vi "LoadArmPressure_old.vi"(8 "error in (no error)":errorcluster, 9 "SHIFTER DATA":T1, 11 "filepath":path) -> (0 "error out":errorcluster)   [LabVIEW 2013, in "main.lvlib"]
uses:
  main.lvlib
  Components/TypeDef - SHIFTER.ctl
  Components/Dependencies.llb/Exit Event Ref.ctl
  New Design/Controls/Reference Cluster.ctl
  <userlib>/_OpenG.lib/file/file.llb/File Exists - Scalar__ogtk.vi
  <vilib>/Utility/file.llb/Read From Spreadsheet File (DBL).vi
  Components/Dependencies.llb/TLB_Dependencies.lvlib
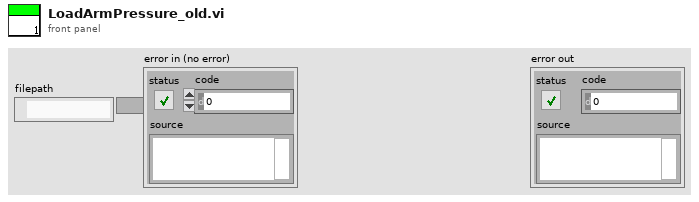
[diagram p1: front panel]
types:
  T1 = typedef "main.lvlib/TypeDef - SHIFTER.ctl" = cluster{"Exit Event":T2, "Terminate Error":errorcluster, "User Parameter Controls":refnum<vi>[], "User Parameters":cluster{"Name":string, "CPR Number":string, "Measuring Type ":string, "Measuring Technique":string, "Measuring Limb":string, "Operator":string, "Doctor":string, "Comment":string, "AdditionalInfo":string, "RightArm":string[][], "LeftArm":string[][], "PalpationRight":string, "PalpationLeft":string, "Puls":dbl, "Temp One":dbl, "Temp Two":dbl, "ActivityBox":bool}, "System Parameters":cluster{"Paper Running?":bool, "GraphSelection":bool, "Date":string, "Active Page":string}, "Data Acquisition":cluster{"Acquisition":bool, "DAQmx Task":refnum<k21>, "DAQmx Error":errorcluster, "Record number":dbl, "RecordPath":path, "AcqDataRef":refnum<vi>, "Duration":timestamp, "Queue":refnum<queue>, "Control?":bool, "RelativeRecordPath":path}, "Reference signal":cluster{"DAQmx  Task ":refnum<k21>, "Monitor":bool, "Events":dbl, "Time":timestamp, "NullEvents":dbl, "RefDataRef":refnum<vi>, "Queue":refnum<queue>}, "Data Process":cluster{"SubpanelRef":refnum<vi>, "ActiveItemTag":string, "Queue":refnum<queue>}, "System Parameter Controls":refnum<vi>[], "Database":cluster{"PatientdataRef":refnum<file>, "PatientdataPath":path, "Blue Pressure":dbl, "Red Pressure":dbl, "ActiveItemTag":string, "Height Adjustment":dbl, "BluePositionArray":dbl[][], "RedPositionArray":dbl[][], "JournalPath":path}, "MWL":cluster{"PatientID":string, "Name":string, "DICOM Info":path, "DICOM Variables":string[], "Worklist":string[][]}, "Control":cluster{"Queue":refnum<queue>, "SignalCluster":cluster{"Pump":bool, "Finger":bool, "Ankle":bool, "Fast Def":bool, "Slow Def":bool, "Init Cal":bool, "Table Pres":bool, "Table":bool}}, "PageMenu":cluster{"VI Reference":refnum<vi>, "Queue":refnum<queue>}, "Profile":cluster{"VI Reference":refnum<vi>, "Queue":refnum<queue>}, "Configuration":cluster{"VI Reference":refnum<vi>, "Queue":refnum<queue>}, "Acquisition":cluster{"VI Reference":refnum<vi>, "Queue":refnum<queue>}, "Data":cluster{"VI Reference":refnum<vi>, "Queue":refnum<queue>}, "Journal":cluster{"VI Reference":refnum<vi>, "Queue":refnum<queue>}, "cRef":T3, "Bluetooth":cluster{"Queue":refnum<queue>, "VI Reference":refnum<vi>}}
  T2 = typedef "main.lvlib/TLB_Dependencies.lvlib/Exit Event Ref.ctl" = refnum<user-event>
  T3 = typedef "main.lvlib/Reference Cluster.ctl" = cluster{"Menu":cluster{"References":cluster{"Stop Acq":refnum<vi>, "MenuExit":refnum<vi>, "MenuStartADC":refnum<vi>, "PersonalInfoString":refnum<vi>, "Profile":refnum<vi>, "Configuration":refnum<vi>, "Acquisition":refnum<vi>, "Data":refnum<vi>, "Journal":refnum<vi>}}, "Profile":cluster{"References":cluster{"Search Patient ID":refnum<vi>, "Name":refnum<vi>, "CommentStr":refnum<vi>, "Listbox Patient ID":refnum<vi>, "ListboxDoctor":refnum<vi>, "ListboxOperator":refnum<vi>, "HospitalName":refnum<vi>, "HospitalDepartment":refnum<vi>, "HospitalAddress":refnum<vi>, "EditHospInfo":refnum<vi>, "Add Patient ID Btn":refnum<vi>, "Query Worklist":refnum<vi>}}, "Configuration":cluster{"References":cluster{"ListboxMeasurementArea":refnum<vi>, "ListboxMeasurementTechnique":refnum<vi>, "ListboxMeasurementMeth":refnum<vi>, "ListboxRightSegmentNr":refnum<vi>, "ListboxLeftSegmentNr":refnum<vi>, "HeightAdjustmentInt":refnum<vi>, "PalpationRight":refnum<vi>, "PalpationLeft":refnum<vi>, "ActivityBox":refnum<vi>}, "New method":cluster{"AddNewMeasurementBtn":refnum<vi>, "Left Time Table":refnum<vi>, "Right Time Table":refnum<vi>}, "Old method":cluster{"LeftArmPressureTable":refnum<vi>, "RightArmPressureTable":refnum<vi>, "SaveArmPressureBtn":refnum<vi>, "Puls":refnum<vi>, "TempTwo":refnum<vi>, "TempOne":refnum<vi>}, "Method":string}, "Acquisition":cluster{"References":cluster{"SegmentAcqString":refnum<vi>, "RingActGraph":refnum<vi>}}, "Data":cluster{"References":cluster{"cmString":refnum<vi>, "AdjustedHeight":refnum<vi>, "Menu":refnum<vi>, "Tangent On/Off":refnum<vi>, "FilterControl":refnum<vi>}}, "Journal":cluster{"References":cluster{"ReportSelection":refnum<vi>, "Data":refnum<vi>, "GenerateReport":refnum<vi>, "Menu":refnum<vi>, "Send To PACS":refnum<vi>}}}
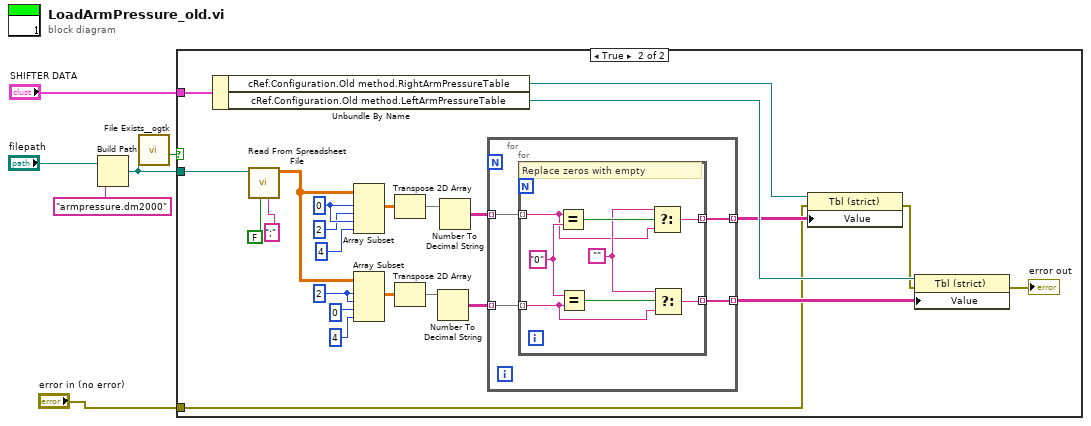
[diagram p0: block diagram]
diagram:
  n1 = Build Path(base path="filepath", name or relative path="armpressure.dm2000") -> (appended path=w2:path)
  n2 = call-poly <userlib>:"File Exists__ogtk.vi"("file path"=w2) -> ("exists"=w4:bool)  [unwired: 6 in, 1 out]
  n3 = case shown="True" w4 {
    tunnel: w2 -> [_ w30]
    tunnel: "SHIFTER DATA" -> [_ w16]
    tunnel: "error in (no error)" -> [_ w8]
    frame False {
    }
    frame True {
      w19 = 2 ("index")
      w27 = 0 ("index")
      n4 = Unbundle By Name(w16) -> ("cRef.Configuration.Old method.RightArmPressureTable"=w15:refnum<vi>, "cRef.Configuration.Old method.LeftArmPressureTable"=w14:refnum<vi>)
      n5 = call-poly <vilib>:"Read From Spreadsheet File.vi"("delimiter (\\t)"=";" ("delimiter (\\t)"), "transpose (no:F)"=FALSE, "file path (dialog if empty)"=w30) -> ("all rows"=w25:dbl[][])  [unwired: 4 in, 4 out]
      n6 = Array Subset(array=w25, index (row)=w27, length (row)=2 ("length"), index (col)=w27, length (col)=4 ("length")) -> (w21:dbl[][])
      n7 = Array Subset(array=w25, index (row)=w19, length (row)=w19, index (col)=0 ("index"), length (col)=4 ("length")) -> (w20:dbl[][])
      n8 = Transpose 2D Array(2D array=w21) -> (transposed array=w18:dbl[][])
      n9 = Transpose 2D Array(2D array=w20) -> (transposed array=w17:dbl[][])
      n10 = Number To Decimal String(number=w17) -> (decimal integer string=w12:string[][])  [unwired: 1 in]
      n11 = Number To Decimal String(number=w18) -> (decimal integer string=w13:string[][])  [unwired: 1 in]
      n12 = for {
        tunnel: w13 -> [w33] mode=indexing
        tunnel: w12 -> [w34] mode=indexing
        tunnel: [w32] -> w11 mode=indexing
        tunnel: [w31] -> w10 mode=indexing
        n13 = for {
          tunnel: w34 -> [w37] mode=indexing
          tunnel: w33 -> [w38] mode=indexing
          tunnel: [w36] -> w32 mode=indexing
          tunnel: [w35] -> w31 mode=indexing
          w39 = ""
          w42 = "0"
          # "Replace zeros with empty"
          n14 = Equal?(x=w38, y=w42) -> (x = y?=w41:bool)
          n15 = Equal?(x=w42, y=w37) -> (x = y?=w40:bool)
          n16 = Select(t=w39, s=w41, f=w38) -> (s? t:f=w36:string)
          n17 = Select(t=w39, s=w40, f=w37) -> (s? t:f=w35:string)
        }
      }
      n18 = property class="Tbl (strict)"(reference=w15, error in=w8, "Value"=w11) -> (error out=w9:errorcluster)  [unwired: 1 out]
      n19 = property class="Tbl (strict)"(reference=w14, error in=w9, "Value"=w10) -> (error out=→"error out":errorcluster)  [unwired: 1 out]
    }
  }
